vi "get source and destination.vi"(6 "regular expression":string="Copying: ", 11 "parh":string) -> (1 "Destination":path, 3 "Source":path)   [LabVIEW 2023]
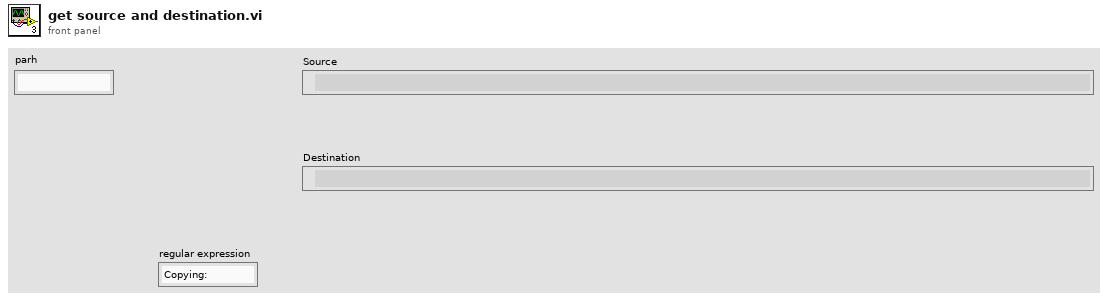
[diagram p1: front panel]
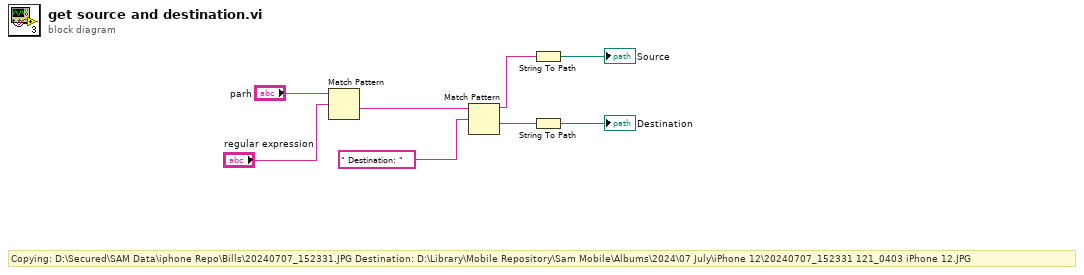
[diagram p0: block diagram]
diagram:
  # "Copying: D:\\Secured\\SAM Data\\iphone Repo\\Bills\\20240707_152331.JPG Destination: D:\\Library\\Mobile Repository\\Sam Mobile\\Albums\\2024\\07 July\\iPhone 12\\20240707_152331 121_0403 iPhone 12.JPG"
  n1 = Match Pattern(string="parh", regular expression="regular expression") -> (after substring=w6:string)  [unwired: 1 in, 3 out]
  n2 = Match Pattern(string=w6, regular expression=" Destination: ") -> (before substring=w4:string, after substring=w1:string)  [unwired: 1 in, 2 out]
  n3 = String To Path(string=w4) -> (path=→"Source":path)
  n4 = String To Path(string=w1) -> (path=→"Destination":path)
